vi "CHP Harm Config.vi"(0 "Instrument Handle In":refnum<k21>, 5 "CHP Config":T2={"Noise Comp Enabled"=0, "Spectrum Power Units"=9, "Integration Bandwidth (Hz)"=1000000.0, "VBW Auto"=1, "VBW (Hz)"=30000.0, "VBW to RBW Ratio"=3.0, "Span (Hz)"=1000000.0, "Sweep Time Interval (s)"=0.001, "Sweep Time Auto"=1, "RBW Filter Type"=1, "RBW (Hz)"=10000.0, "RBW Auto"=1, "Averaging Enabled"=0, "Averaging Count"=10, "Averaging Type"=0, "Measurement Interval (s)"=0.0001, "Preamp Enabled"=0, "Preselector Enabled"=0} {"Preselector Enabled" items=["Disabled", "Enabled"]; "Preamp Enabled" items=["Disabled"=0, "Enabled"=1, "Automatic"=3]; "Measurement Interval (s)" format="%.3p"; "Averaging Type" items=["RMS", "Log", "Scalar", "Max", "Min"]; "Averaging Enabled" items=["False", "True"]; "RBW Auto" items=["False", "True"]; "RBW (Hz)" format="%.3p"; "RBW Filter Type" items=["FFT Based", "Gaussian", "Flat"]; "Sweep Time Auto" items=["False", "True"]; "Sweep Time Interval (s)" format="%.2p"; "Span (Hz)" format="%.3p"; "VBW to RBW Ratio" format="%#.6f"; "VBW (Hz)" format="%.3p"; "VBW Auto" items=["False", "True"]; "Integration Bandwidth (Hz)" format="%.3p"; "Spectrum Power Units" items=["dBm", "dBm/Hz", "dBW", "dBV", "dBmV", "dBuV", "W", "Volts", "Volts Squared", "Reference Level Units"]; "Noise Comp Enabled" items=["False", "True"]}, 7 "Harmonics Config":T1={"Harmonic to Measure"=0.0, "Fundamental Frequency (Hz)"=0.0, "RF Attenuation"=0.0, "RF Attenuation Auto"=1} {"RF Attenuation Auto" items=["False", "True"]}, 11 "error in (no error)":errorcluster) -> (4 "Instrument Handle Out":refnum<k21>, 6 "Reference Level (dBm)":dbl format="%.2f", 15 "error out":errorcluster)   [LabVIEW 2018, in "RFmxSpecAn.lvlib"]
uses:
  RFmxSpecAn.lvlib
  Typedefs/CHP Configuration.ctl
  Typedefs/Harmonics Config.ctl
  <vilib>/RFmx/SpecAn/mx/RFmxSpecAn.llb/RFmxSpecAn Select Measurement (Multiple).vi
  <resource>/objmgr/RFmxInstr.rc
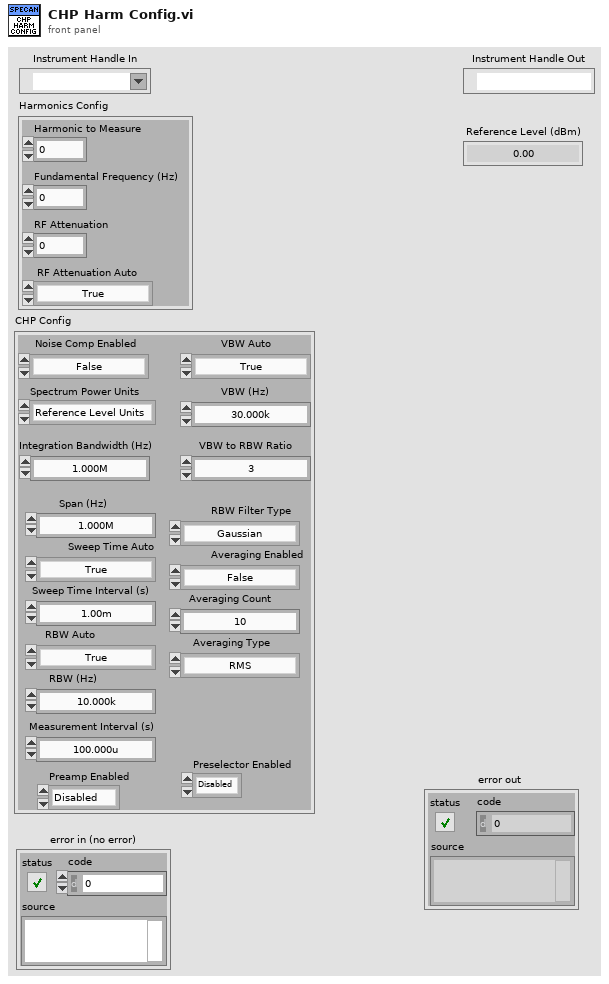
[diagram p1: front panel]
types:
  T1 = typedef "RFmxSpecAn.lvlib/Harmonics Config.ctl" = cluster{"Harmonic to Measure":dbl, "Fundamental Frequency (Hz)":dbl, "RF Attenuation":dbl, "RF Attenuation Auto":i32}
  T2 = typedef "RFmxSpecAn.lvlib/CHP Configuration.ctl" = cluster{"Noise Comp Enabled":i32, "Spectrum Power Units":i32, "Integration Bandwidth (Hz)":dbl, "VBW Auto":i32, "VBW (Hz)":dbl, "VBW to RBW Ratio":dbl, "Span (Hz)":dbl, "Sweep Time Interval (s)":dbl, "Sweep Time Auto":i32, "RBW Filter Type":i32, "RBW (Hz)":dbl, "RBW Auto":i32, "Averaging Enabled":i32, "Averaging Count":i32, "Averaging Type":i32, "Measurement Interval (s)":dbl, "Preamp Enabled":i32, "Preselector Enabled":i32}
  T3 = enum16{"ACP", "CCDF", "CHP", "FCnt", "Harmonics", "OBW", "SEM", "Spectrum", "Spur", "TXP", "AMPM", "DPD", "IQ", "IM", "NF", "PhaseNoise"}[]
  T4 = cluster{"Noise Comp Enabled":dbl, "Spectrum Power Units":dbl, "Integration Bandwidth (Hz)":dbl, "VBW Auto":dbl, "VBW (Hz)":dbl, "VBW to RBW Ratio":dbl, "Span (Hz)":dbl, "Sweep Time Interval (s)":dbl, "Sweep Time Auto":dbl, "RBW Filter Type":dbl, "RBW (Hz)":dbl, "RBW Auto":dbl, "Averaging Enabled":dbl, "Averaging Count":dbl, "Averaging Type":dbl, "Measurement Interval (s)":dbl, "Preamp Enabled":dbl, "Preselector Enabled":dbl}
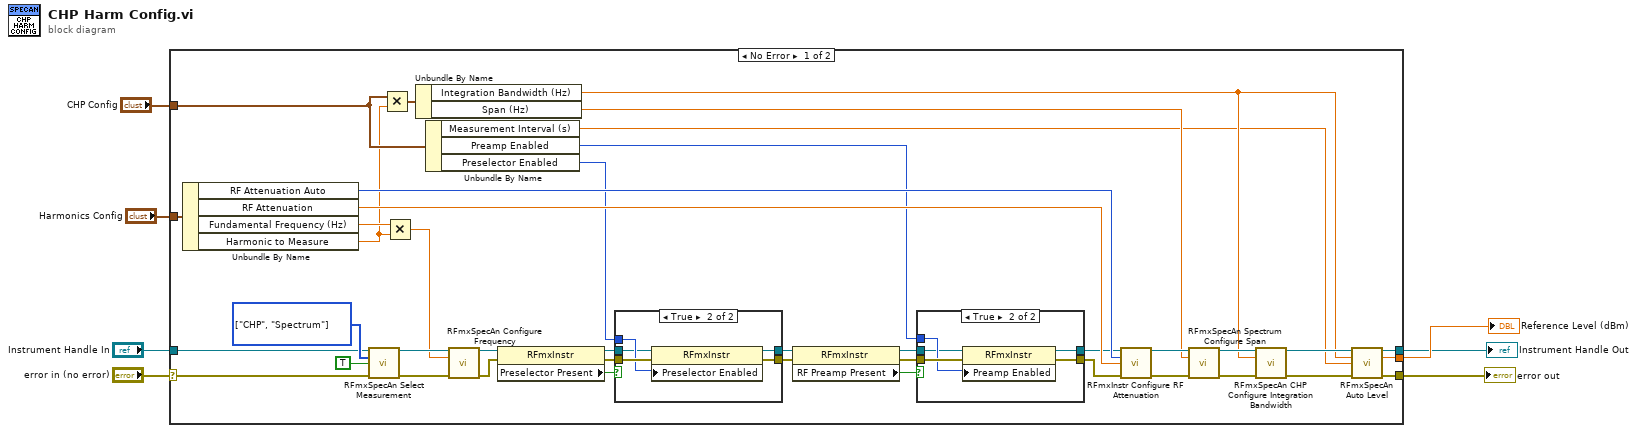
[diagram p0: block diagram]
diagram:
  n1 = case shown="No Error" "error in (no error)" {
    selector: "error in (no error)" -> [w26 w62]
    tunnel: "Harmonics Config" -> [w36 _]
    tunnel: "CHP Config" -> [w34 _]
    tunnel: [w28 _] -> w5
    tunnel: [w27 w63] -> w4
    tunnel: "Instrument Handle In" -> [w25 w63]
    tunnel: [w24 w62] -> w1
    frame No Error {
      w41 = T3 [enum."CHP", enum."Spectrum"] items=["ACP", "CCDF", "CHP", "FCnt", "Harmonics", "OBW", "SEM", "Spectrum", "Spur", "TXP", "AMPM", "DPD", "IQ", "IM", "NF", "PhaseNoise"]
      n2 = Unbundle By Name(w36) -> ("RF Attenuation Auto"=w23:i32, "RF Attenuation"=w32:dbl, "Fundamental Frequency (Hz)"=w35:dbl, "Harmonic to Measure"=w22:dbl)
      n3 = call-poly <vilib>:"RFmxSpecAn Select Measurement.vi"("Instrument Handle In"=w25, "Measurements"=w41, "Enable All Traces"=TRUE, "error in (no error)"=w26) -> ("Instrument Handle Out"=w38:refnum<k21>, "error out"=w39:errorcluster)  [unwired: 10 in]
      n4 = Multiply(x=w34, y=w22) -> (x*y=w37:T4)
      n5 = Multiply(x=w35, y=w22) -> (x*y=w33:dbl)
      n6 = Unbundle By Name(w37) -> ("Integration Bandwidth (Hz)"=w30:dbl, "Span (Hz)"=w31:dbl)
      n7 = Unbundle By Name(w34) -> ("Measurement Interval (s)"=w29:dbl, "Preamp Enabled"=w9:i32, "Preselector Enabled"=w8:i32)
      n8 = call <vilib>:"RFmxSpecAn Configure Frequency.vi"("Instrument Handle In"=w38, "Center Frequency (Hz)"=w33, "error in (no error)"=w39) -> ("Instrument Handle Out"=w13:refnum<k21>, "error out"=w12:errorcluster)  [unwired: 11 in]
      n9 = property class="RFmxInstr"(reference=w13, error in=w12) -> (reference out=w16:refnum<k21>, error out=w15:errorcluster, "Preselector Present"=w14:bool)
      n10 = case shown="True" w14 {
        tunnel: w15 -> [w48 w54]
        tunnel: w8 -> [_ w53]
        tunnel: w16 -> [w49 w52]
        tunnel: [w48 w51] -> w17
        tunnel: [w49 w50] -> w18
        frame False {
        }
        frame True {
          n11 = property class="RFmxInstr"(reference=w52, error in=w54, "Preselector Enabled"=w53) -> (reference out=w50:refnum<k21>, error out=w51:errorcluster)
        }
      }
      n12 = property class="RFmxInstr"(reference=w18, error in=w17) -> (reference out=w21:refnum<k21>, error out=w20:errorcluster, "RF Preamp Present"=w19:bool)
      n13 = case shown="True" w19 {
        tunnel: w20 -> [w55 w61]
        tunnel: w9 -> [_ w60]
        tunnel: w21 -> [w56 w59]
        tunnel: [w55 w58] -> w10
        tunnel: [w56 w57] -> w11
        frame False {
        }
        frame True {
          n14 = property class="RFmxInstr"(reference=w59, error in=w61, "Preamp Enabled"=w60) -> (reference out=w57:refnum<k21>, error out=w58:errorcluster)
        }
      }
      n15 = call <vilib>:"RFmxInstr Configure RF Attenuation.vi"("Instrument Handle In"=w11, "RF Attenuation Auto"=w23, "RF Attenuation (dB)"=w32, "error in (no error)"=w10) -> ("Instrument Handle Out"=w43:refnum<k21>, "error out"=w42:errorcluster)  [unwired: 10 in]
      n16 = call <vilib>:"RFmxSpecAn Spectrum Configure Span.vi"("Instrument Handle In"=w43, "Span (Hz)"=w31, "error in (no error)"=w42) -> ("Instrument Handle Out"=w45:refnum<k21>, "error out"=w44:errorcluster)  [unwired: 11 in]
      n17 = call <vilib>:"RFmxSpecAn CHP Configure Integration Bandwidth.vi"("Instrument Handle In"=w45, "Integration Bandwidth (Hz)"=w30, "error in (no error)"=w44) -> ("Instrument Handle Out"=w47:refnum<k21>, "error out"=w46:errorcluster)  [unwired: 11 in]
      n18 = call <vilib>:"RFmxSpecAn Auto Level.vi"("Instrument Handle In"=w47, "Bandwidth (Hz)"=w30, "Measurement Interval (s)"=w29, "error in (no error)"=w46) -> ("Instrument Handle Out"=w27:refnum<k21>, "Reference Level (dBm)"=w28:dbl, "error out"=w24:errorcluster)  [unwired: 9 in]
    }
    frame Error {
    }
  }
  "Reference Level (dBm)" <- w5
  "Instrument Handle Out" <- w4
  "error out" <- w1
